vi "InfobarSection.vi"(8 "Infobar In":string, 11 "Section":string) -> (0 "Infobar Out":string)   [LabVIEW 2016]
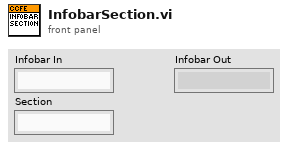
[diagram p1: front panel]
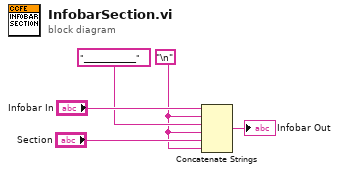
[diagram p0: block diagram]
diagram:
  w2 = "\n"
  n1 = Concatenate Strings("Infobar In", w2, "_____________", w2, "Section", w2) -> (→"Infobar Out":string)
